vi "Get Menu CMD.vi"(11 "Front Panel Menu in":refnum<class "Front Panel Menu.lvclass">) -> (0 "Item Path":string, 2 "Itme Tag":string, 3 "Front Panel Menu out":refnum<class "Front Panel Menu.lvclass">)   [LabVIEW 2024, in "Front Panel Menu.lvclass"]
uses:
  Front Panel Menu.lvclass
  Front Panel Menu.lvclass/Front Panel Menu.ctl
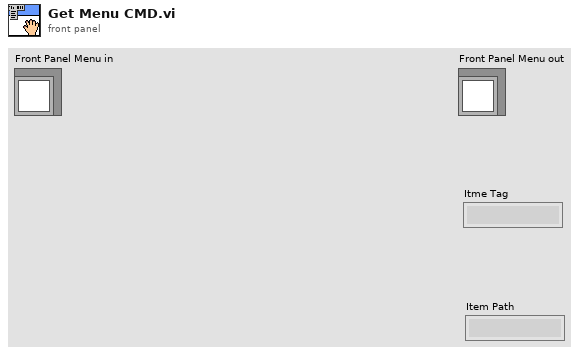
[diagram p1: front panel]
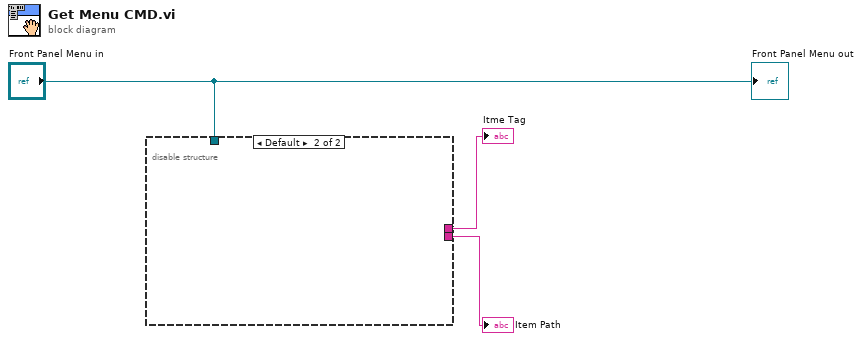
[diagram p0: block diagram]
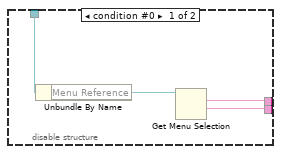
[diagram p2: hidden frame]
diagram:
  n1 = disable-structure shown="Default" {
    disable-tunnel: "Front Panel Menu in" -> [w4 _]
    disable-tunnel: [w6 _] -> w2
    disable-tunnel: [w5 _] -> w1
    frame condition #0 {
      n2 = Unbundle By Name(w4) -> ("Menu Reference"=w7:refnum<k9>)
      n3 = Get Menu Selection(0:w7) -> (6:w6:string, 7:w5:string)  [unwired: 3 in, 3 out]
    }
    frame condition #1 (active) {
    }
  }
  "Itme Tag" <- w2
  "Item Path" <- w1
  "Front Panel Menu out" <- "Front Panel Menu in"
